vi "CreateGenerateMessage.vi"(8 "error in (no error)":errorcluster, 11 "Message in":T1) -> (0 "error out":errorcluster, 3 "Message out":T1)   [LabVIEW 2017, in "MessageGen.lvlib"]
uses:
  <vilib>/addons/InsightCM/MessageBus/CodeGen/MessageGen.lvlib
  <vilib>/addons/InsightCM/MessageBus/CodeGen/controls/MessageData.ctl
  <vilib>/addons/InsightCM/MessageBus/CodeGen/controls/MessageType.ctl
  <vilib>/addons/InsightCM/MessageBus/CodeGen/controls/Parameter.ctl
  <vilib>/addons/InsightCM/MessageBus/CodeGen/controls/ParameterType.ctl
  <vilib>/LabVIEW Icon API/API_Text.ctl
  <vilib>/LabVIEW Icon API/LabVIEW Icon API.lvlib
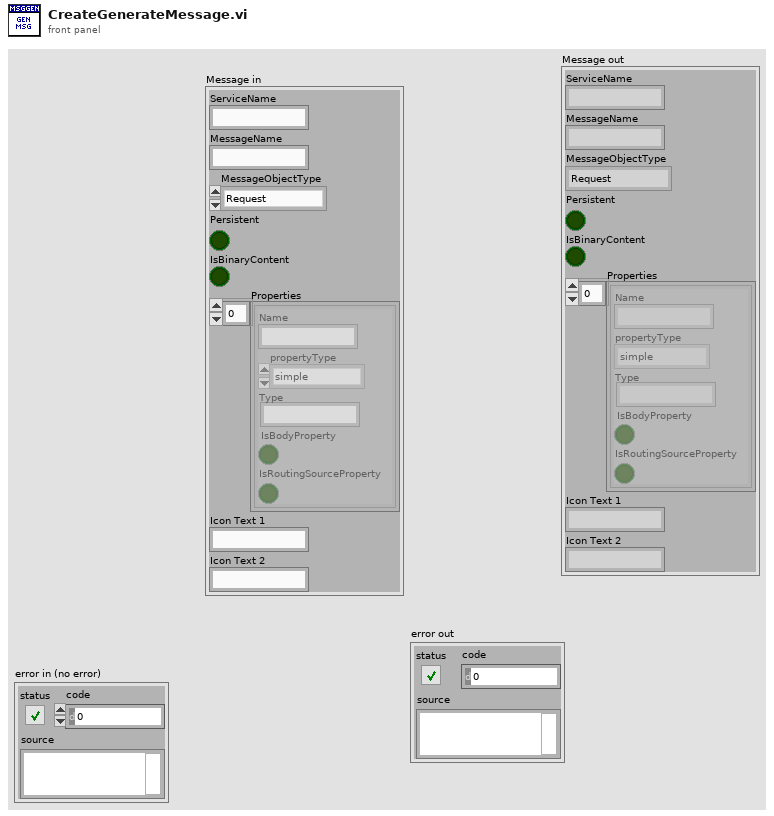
[diagram p1: front panel]
types:
  T1 = typedef "MessageGen.lvlib/MessageData.ctl" = cluster{"ServiceName":string, "MessageName":string, "MessageObjectType":T2, "Persistent":bool, "IsBinaryContent":bool, "Properties":T3[], "Icon Text 1":string, "Icon Text 2":string}
  T2 = typedef "MessageGen.lvlib/MessageType.ctl" = enum16{"Request", "Response", "Broadcast", "RoutedMessage"}
  T3 = typedef "MessageGen.lvlib/Parameter.ctl" = cluster{"Name":string, "propertyType":T4, "Type":string, "IsBodyProperty":bool, "IsRoutingSourceProperty":bool}
  T4 = typedef "MessageGen.lvlib/ParameterType.ctl" = enum16{"simple", "bytearray", "dateTime", "list", "map", "object"}
  T5 = typedef "LabVIEW Icon API.lvlib/API_Text.ctl" = cluster{"Line 1 text":string, "Line 2 text":string, "Line 3 text":string, "Line 4 text":string}
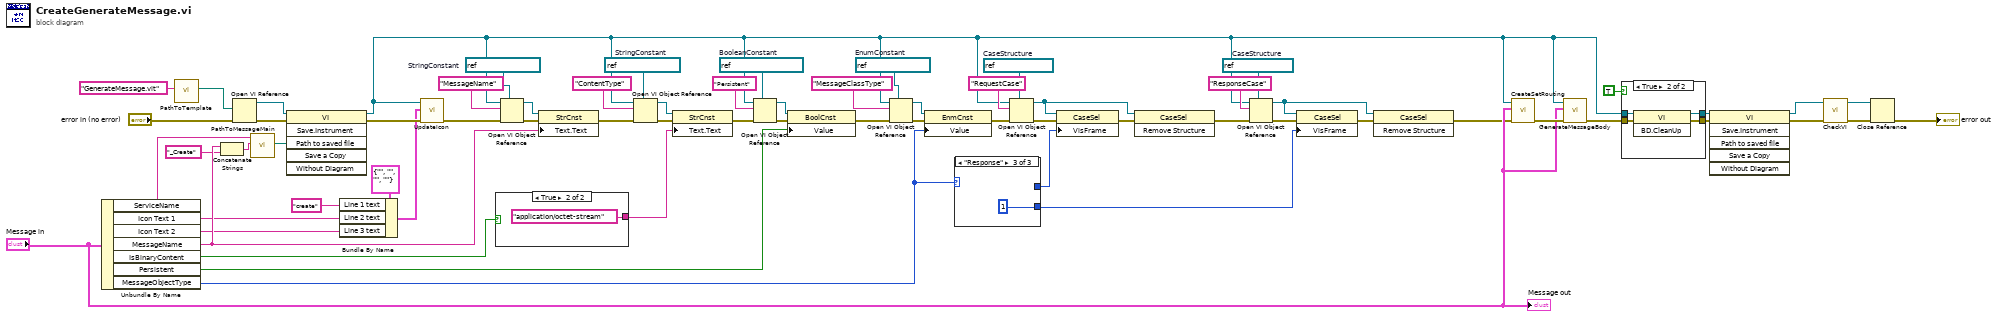
[diagram p0: block diagram]
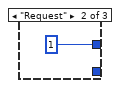
[diagram p4: hidden frame]
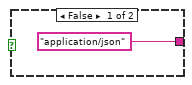
[diagram p5: hidden frame]
diagram:
  w10 = refnum<vi> refnum  # CaseStructure
  w22 = refnum<vi> refnum  # CaseStructure
  w40 = refnum<vi> refnum  # EnumConstant
  w52 = refnum<vi> refnum  # BooleanConstant
  w57 = refnum<vi> refnum  # StringConstant
  w62 = refnum<vi> refnum  # StringConstant
  n1 = Unbundle By Name("Message in") -> ("ServiceName"=w30:string, "Icon Text 1"=w13:string, "Icon Text 2"=w12:string, "MessageName"=w17:string, "IsBinaryContent"=w44:bool, "Persistent"=w43:bool, "MessageObjectType"=w20:T2)
  n2 = call <vilib>:"PathToTemplate.vi"("TemplateName"="GenerateMessage.vit") -> ("Path"=w47:path)  [unwired: 10 in]
  n3 = Concatenate Strings(w17, "_Create" ("string")) -> (w31:string)
  n4 = Open VI Reference(vi path=w47, error in (no error)="error in (no error)") -> (vi reference=w64:refnum<vi>, error out=w65:errorcluster)  [unwired: 4 in]
  n5 = call <vilib>:"PathToMessageMain.vi"("VIName"=w31, "Service"=w30) -> ("Path"=w29:path)  [unwired: 9 in]
  n6 = invoke class="VI" method="Save.Instrument"(reference=w64, error in=w65, "Path to saved file"=w29) -> (reference out=w2:refnum<vi>, error out=w46:errorcluster)  [unwired: 3 in, 4 out]
  n7 = Bundle By Name(cluster=T5 {"Line 1 text"="", "Line 2 text"="", "Line 3 text"="", "Line 4 text"=""} ("Text"), "Line 1 text"="create" ("method"), "Line 2 text"=w13, "Line 3 text"=w12) -> (w11:T5)
  n8 = call <vilib>:"UpdateIcon.vi"("error in (no error)"=w46, "Text"=w11, "VI Refnum in"=w2) -> ("error out"=w45:errorcluster)  [unwired: 7 in, 1 out]
  n9 = case shown="True" w44 {
    tunnel: ["application/json" "application/octet-stream"] -> w54
    frame False {
    }
    frame True {
    }
  }
  n10 = Open VI Object Reference(7:w62, 8:w45, 10:"MessageName" ("name/order"), 11:w2) -> (0:w60:errorcluster, 3:w61:refnum<vi>)
  n11 = property class="StrCnst"(reference=w61, error in=w60, "Text.Text"=w17) -> (error out=w55:errorcluster)  [unwired: 1 out]
  n12 = Open VI Object Reference(7:w57, 8:w55, 10:"ContentType" ("name/order"), 11:w2) -> (0:w59:errorcluster, 3:w58:refnum<vi>)
  n13 = property class="StrCnst"(reference=w58, error in=w59, "Text.Text"=w54) -> (error out=w49:errorcluster)  [unwired: 1 out]
  n14 = Open VI Object Reference(7:w52, 8:w49, 10:"Persistent" ("name/order"), 11:w2) -> (0:w50:errorcluster, 3:w51:refnum<vi>)
  n15 = property class="BoolCnst"(reference=w51, error in=w50, "Value"=w43) -> (error out=w39:errorcluster)  [unwired: 1 out]
  n16 = Open VI Object Reference(7:w40, 8:w39, 10:"MessageClassType" ("name/order"), 11:w2) -> (0:w42:errorcluster, 3:w41:refnum<vi>)
  n17 = property class="EnmCnst"(reference=w41, error in=w42, "Value"=w20) -> (error out=w21:errorcluster)  [unwired: 1 out]
  n18 = case shown="\"Response\"" w20 {
    tunnel: [_ u32 1 _] -> w19
    tunnel: [_ _ u32 1] -> w3
    frame "Broadcast", "RoutedMessage" {
    }
    frame "Request" {
    }
    frame "Response" {
    }
  }
  n19 = Open VI Object Reference(7:w22, 8:w21, 10:"RequestCase" ("name/order"), 11:w2) -> (0:w26:errorcluster, 3:w25:refnum<vi>)
  n20 = property class="CaseSel"(reference=w25, error in=w26, "VisFrame"=w19) -> (error out=w24:errorcluster)  [unwired: 1 out]
  n21 = invoke class="CaseSel" method="Remove Structure"(reference=w25, error in=w24) -> (error out=w6:errorcluster)  [unwired: 1 in, 2 out]
  n22 = Open VI Object Reference(7:w10, 8:w6, 10:"ResponseCase" ("name/order"), 11:w2) -> (0:w7:errorcluster, 3:w8:refnum<vi>)
  n23 = property class="CaseSel"(reference=w8, error in=w7, "VisFrame"=w3) -> (error out=w9:errorcluster)  [unwired: 1 out]
  n24 = invoke class="CaseSel" method="Remove Structure"(reference=w8, error in=w9) -> (error out=w5:errorcluster)  [unwired: 1 in, 2 out]
  n25 = call <vilib>:"CreateSetRouting.vi"("error in (no error)"=w5, "Message in"="Message in", "VI reference"=w2) -> ("error out"=w33:errorcluster)  [unwired: 8 in]
  n26 = call <vilib>:"GenerateMessageBody.vi"("error in (no error)"=w33, "Message"="Message in", "VI reference"=w2) -> ("error out"=w1:errorcluster)  [unwired: 8 in]
  n27 = case shown="True" TRUE {
    tunnel: w1 -> [w72 w77]
    tunnel: [w72 w76] -> w28
    tunnel: w2 -> [w73 w75]
    tunnel: [w73 w74] -> w27
    frame False {
    }
    frame True {
      n28 = invoke class="VI" method="BD.CleanUp"(reference=w75, error in=w77) -> (reference out=w74:refnum<vi>, error out=w76:errorcluster)  [unwired: 1 in, 1 out]
    }
  }
  n29 = invoke class="VI" method="Save.Instrument"(reference=w27, error in=w28) -> (reference out=w37:refnum<vi>, error out=w35:errorcluster)  [unwired: 4 in, 4 out]
  n30 = call <vilib>:"CheckVI.vi"("error in (no error)"=w35, "VI ref"=w37) -> ("error out"=w34:errorcluster, "VI ref out"=w36:refnum<vi>)  [unwired: 8 in]
  n31 = Close Reference(reference=w36, error in (no error)=w34) -> (error out=→"error out":errorcluster)
  "Message out" <- "Message in"
